vi "RTDAQ (1).vi"(8 "error in (no error)":errorcluster) -> (0 "error out":errorcluster)   [LabVIEW 2017]
doc: "Reads actual data from inputs for full systems runs or virtual data from SimulatedDataGLOBAL.vi for testing. Converts the data into an array of double precision values and sends it to the user, HostMain.vi, and RTControl.vi."
uses:
  Sensors/SimulatedSensorsGLOBAL.vi
  LoopPeriodGLOBAL.vi
  RTControl/StopGLOBAL.vi
panel:
  out "size(s)":i32
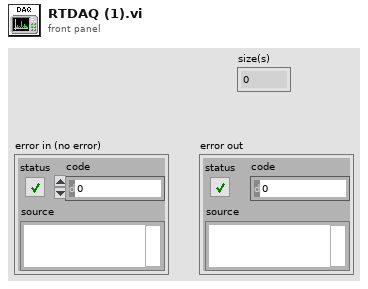
[diagram p1: front panel]
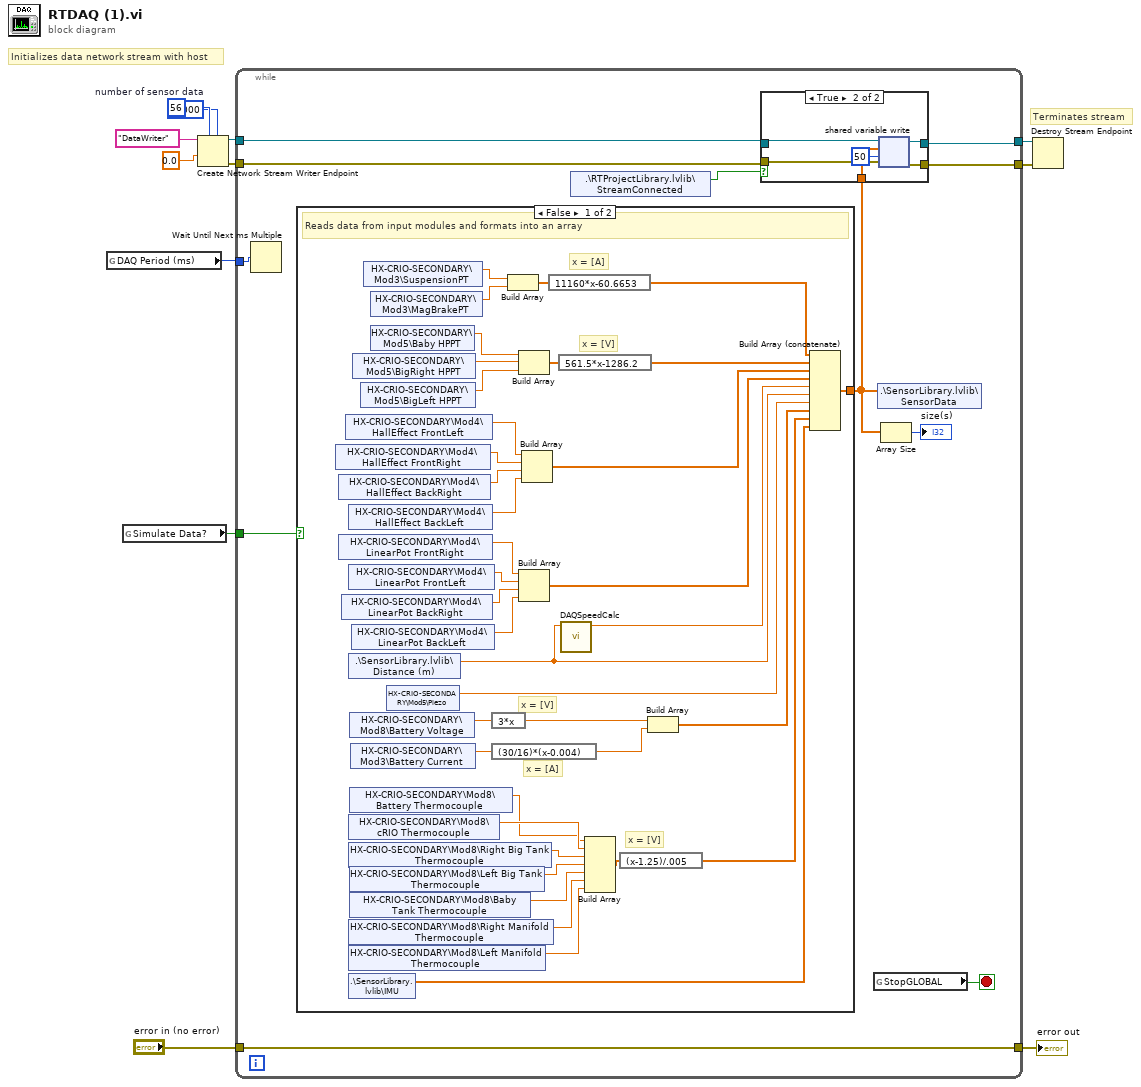
[diagram p0: block diagram]
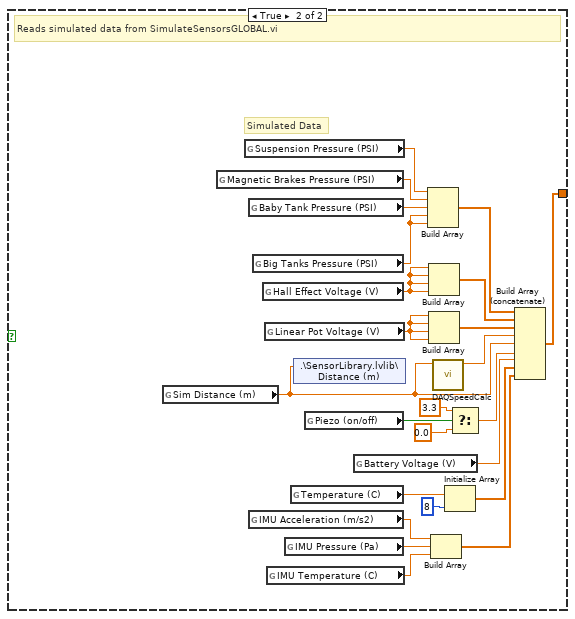
[diagram p3: hidden frame]
diagram:
  w12 = 56  # number of sensor data
  # "Terminates stream"
  # "Initializes data network stream with host"
  n1 = global read "LoopPeriodGLOBAL.vi" "DAQ Period (ms)"() -> (w2:u32)
  n2 = global read "SimulatedSensorsGLOBAL.vi" "Simulate Data?"() -> (w5:bool)
  n3 = Create Network Stream Writer Endpoint(5:10000 ("timeout in ms (-1)"), 7:w12, 9:0.0, 11:"DataWriter" ("writer name")) -> (0:w8:errorcluster, 3:w9:refnum<k21>)  [unwired: 3 in]
  n4 = while {
    tunnel: w2 -> [w23]
    tunnel: w9 -> [w16]
    tunnel: w8 -> [w17]
    tunnel: [w22] -> w7
    tunnel: [w21] -> w6
    tunnel: w5 -> [w19]
    tunnel: "error in (no error)" -> [w18]
    tunnel: [w18] -> w3
    stop <- w20 stop-if-true
    n5 = Wait Until Next ms Multiple(millisecond multiple=w23) -> ()  [unwired: 1 out]
    n6 = case shown="False" w19 {
      tunnel: [w56 w93] -> w15
      frame False {
        # "x = [A]"
        # "x = [A]"
        # "x = [V]"
        # "x = [V]"
        # "x = [V]"
        # "Reads data from input modules and formats into an array"
        n7 = shared-variable "HX-CRIO-SECONDARY\\Mod4\\HallEffect FrontRight"() -> (w65:dbl)  [unwired: 1 in, 1 out]
        n8 = shared-variable "HX-CRIO-SECONDARY\\Mod4\\HallEffect BackRight"() -> (w64:dbl)  [unwired: 1 in, 1 out]
        n9 = shared-variable "HX-CRIO-SECONDARY\\Mod4\\LinearPot FrontRight"() -> (w66:dbl)  [unwired: 1 in, 1 out]
        n10 = shared-variable "HX-CRIO-SECONDARY\\Mod4\\LinearPot BackRight"() -> (w61:dbl)  [unwired: 1 in, 1 out]
        n11 = shared-variable "HX-CRIO-SECONDARY\\Mod4\\HallEffect FrontLeft"() -> (w68:dbl)  [unwired: 1 in, 1 out]
        n12 = shared-variable "HX-CRIO-SECONDARY\\Mod4\\HallEffect BackLeft"() -> (w63:dbl)  [unwired: 1 in, 1 out]
        n13 = shared-variable "HX-CRIO-SECONDARY\\Mod4\\LinearPot FrontLeft"() -> (w62:dbl)  [unwired: 1 in, 1 out]
        n14 = shared-variable ".\\SensorLibrary.lvlib\\Distance (m)"() -> (w41:dbl)  [unwired: 1 in, 1 out]
        n15 = shared-variable "HX-CRIO-SECONDARY\\Mod8\\cRIO Thermocouple"() -> (w39:dbl)  [unwired: 1 in, 1 out]
        n16 = shared-variable "HX-CRIO-SECONDARY\\Mod8\\Right Big Tank Thermocouple"() -> (w53:dbl)  [unwired: 1 in, 1 out]
        n17 = shared-variable "HX-CRIO-SECONDARY\\Mod8\\Right Manifold Thermocouple"() -> (w50:dbl)  [unwired: 1 in, 1 out]
        n18 = shared-variable "HX-CRIO-SECONDARY\\Mod8\\Left Manifold Thermocouple"() -> (w49:dbl)  [unwired: 1 in, 1 out]
        n19 = shared-variable ".\\SensorLibrary.lvlib\\IMU"() -> (w46:dbl[])  [unwired: 1 in, 1 out]
        n20 = shared-variable "HX-CRIO-SECONDARY\\Mod8\\Battery Voltage"() -> (w55:dbl)  [unwired: 1 in, 1 out]
        n21 = shared-variable "HX-CRIO-SECONDARY\\Mod8\\Battery Thermocouple"() -> (w38:dbl)  [unwired: 1 in, 1 out]
        n22 = shared-variable "HX-CRIO-SECONDARY\\Mod8\\Left Big Tank Thermocouple"() -> (w52:dbl)  [unwired: 1 in, 1 out]
        n23 = shared-variable "HX-CRIO-SECONDARY\\Mod8\\Baby Tank Thermocouple"() -> (w51:dbl)  [unwired: 1 in, 1 out]
        n24 = shared-variable "HX-CRIO-SECONDARY\\Mod3\\Battery Current"() -> (w37:dbl)  [unwired: 1 in, 1 out]
        n25 = shared-variable "HX-CRIO-SECONDARY\\Mod4\\LinearPot BackLeft"() -> (w60:dbl)  [unwired: 1 in, 1 out]
        n26 = shared-variable "HX-CRIO-SECONDARY\\Mod5\\BigRight HPPT"() -> (w44:dbl)  [unwired: 1 in, 1 out]
        n27 = shared-variable "HX-CRIO-SECONDARY\\Mod5\\BigLeft HPPT"() -> (w45:dbl)  [unwired: 1 in, 1 out]
        n28 = shared-variable "HX-CRIO-SECONDARY\\Mod3\\SuspensionPT"() -> (w34:dbl)  [unwired: 1 in, 1 out]
        n29 = shared-variable "HX-CRIO-SECONDARY\\Mod3\\MagBrakePT"() -> (w33:dbl)  [unwired: 1 in, 1 out]
        n30 = shared-variable "HX-CRIO-SECONDARY\\Mod5\\Baby HPPT"() -> (w43:dbl)  [unwired: 1 in, 1 out]
        n31 = shared-variable "HX-CRIO-SECONDARY\\Mod5\\Piezo"() -> (w42:dbl)  [unwired: 1 in, 1 out]
        n32 = expression code="3*x"(w55) -> (w54:dbl)
        n33 = expression code="(30/16)*(x-0.004)"(w37) -> (w35:dbl)
        n34 = Build Array(w34, w33) -> (w32:dbl[])
        n35 = Build Array(w43, w44, w45) -> (w69:dbl[])
        n36 = Build Array(w66, w62, w61, w60) -> (w57:dbl[])
        n37 = Build Array(w68, w65, w64, w63) -> (w67:dbl[])
        n38 = expression code="11160*x-60.6653"(w32) -> (w59:dbl[])
        n39 = expression code="561.5*x-1286.2"(w69) -> (w58:dbl[])
        n40 = call "DAQSpeedCalc.vi"("Distance"=w41) -> ("Speed"=w40:dbl)  [unwired: 10 in]
        n41 = Build Array(w38, w39, w53, w52, w51, w50, w49) -> (w48:dbl[])
        n42 = expression code="(x-1.25)/.005"(w48) -> (w47:dbl[])
        n43 = Build Array(w54, w35) -> (w36:dbl[])
        n44 = Build Array (concatenate)(w59, w58, w67, w57, w40, w41, w42, w36, w47, w46) -> (w56:dbl[])
      }
      frame True {
        # "Simulated Data"
        # "Reads simulated data from SimulateSensorsGLOBAL.vi"
        n45 = global read "SimulatedSensorsGLOBAL.vi" "Sim Distance (m)"() -> (w71:dbl)
        n46 = global read "SimulatedSensorsGLOBAL.vi" "Magnetic Brakes Pressure (PSI)"() -> (w82:dbl)
        n47 = global read "SimulatedSensorsGLOBAL.vi" "Suspension Pressure (PSI)"() -> (w81:dbl)
        n48 = global read "SimulatedSensorsGLOBAL.vi" "Baby Tank Pressure (PSI)"() -> (w84:dbl)
        n49 = global read "SimulatedSensorsGLOBAL.vi" "IMU Acceleration (m/s2)"() -> (w79:dbl)
        n50 = global read "SimulatedSensorsGLOBAL.vi" "Big Tanks Pressure (PSI)"() -> (w74:dbl)
        n51 = global read "SimulatedSensorsGLOBAL.vi" "Hall Effect Voltage (V)"() -> (w90:dbl)
        n52 = global read "SimulatedSensorsGLOBAL.vi" "Linear Pot Voltage (V)"() -> (w91:dbl)
        n53 = global read "SimulatedSensorsGLOBAL.vi" "IMU Temperature (C)"() -> (w92:dbl)
        n54 = global read "SimulatedSensorsGLOBAL.vi" "IMU Pressure (Pa)"() -> (w80:dbl)
        n55 = global read "SimulatedSensorsGLOBAL.vi" "Temperature (C)"() -> (w77:dbl)
        n56 = shared-variable ".\\SensorLibrary.lvlib\\Distance (m)"(w71) -> ()  [unwired: 1 in, 1 out]
        n57 = global read "SimulatedSensorsGLOBAL.vi" "Piezo (on/off)"() -> (w87:bool)
        n58 = global read "SimulatedSensorsGLOBAL.vi" "Battery Voltage (V)"() -> (w72:dbl)
        n59 = Build Array(w81, w82, w84, w74, w74) -> (w83:dbl[])
        n60 = Build Array(w90, w90, w90, w90) -> (w88:dbl[])
        n61 = Build Array(w91, w91, w91, w91) -> (w89:dbl[])
        n62 = Build Array(w79, w80, w92) -> (w78:dbl[])
        n63 = call "DAQSpeedCalc.vi"("Distance"=w71) -> ("Speed"=w70:dbl)  [unwired: 10 in]
        n64 = Initialize Array(w77, 8 ("dimension size")) -> (w75:dbl[])
        n65 = Select(t=3.3, s=w87, f=0.0) -> (s? t:f=w73:dbl)
        n66 = Build Array (concatenate)(w83, w88, w89, w70, w71, w73, w72, w75, w78) -> (w93:dbl[])
      }
    }
    n67 = shared-variable ".\\RTProjectLibrary.lvlib\\StreamConnected"() -> (w13:bool)  [unwired: 1 in, 1 out]
    n68 = case shown="True" w13 {
      tunnel: [w25 w31] -> w22
      tunnel: [w24 w30] -> w21
      tunnel: w15 -> [_ w29]
      tunnel: w17 -> [w24 w28]
      tunnel: w16 -> [w25 w27]
      frame False {
      }
      frame True {
        n69 = shared-variable-write(w27, w28, w29, 50 ("timeout ms (-1)")) -> (w31:refnum<k21>, w30:errorcluster)  [unwired: 1 out]
      }
    }
    n70 = global read "StopGLOBAL.vi" "StopGLOBAL"() -> (w20:bool)
    n71 = shared-variable ".\\SensorLibrary.lvlib\\SensorData"(w15) -> ()  [unwired: 1 in, 1 out]
    n72 = Array Size(array=w15) -> (size(s)=→"size(s)":i32)
  }
  "error out" <- w3
  n73 = Destroy Stream Endpoint(8:w6, 11:w7) -> ()  [unwired: 1 out]
